vi "CountConfig.vi"(7 "Cal (F)/Acq (T) Counters":bool, 10 "Machine Type":enum16{"Hitachi", "B&K 3535", "B&K Hawk"}(ring), 11 "pulse delay  (cycles)":i16=1 caption="pulse delay (cycles)") -> (2 "task out":refnum<k21>)   [LabVIEW 2022 SP3]
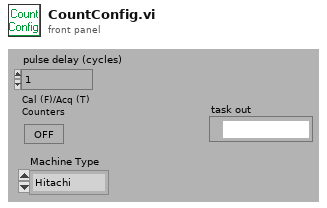
[diagram p1: front panel]
types:
  T1 = enum16{"gate on rising edge", "gate on falling edge"}
  T2 = enum16{"count on rising edge", "count on falling edge"}
  T3 = enum16{"arm on rising edge", "arm on falling edge"}
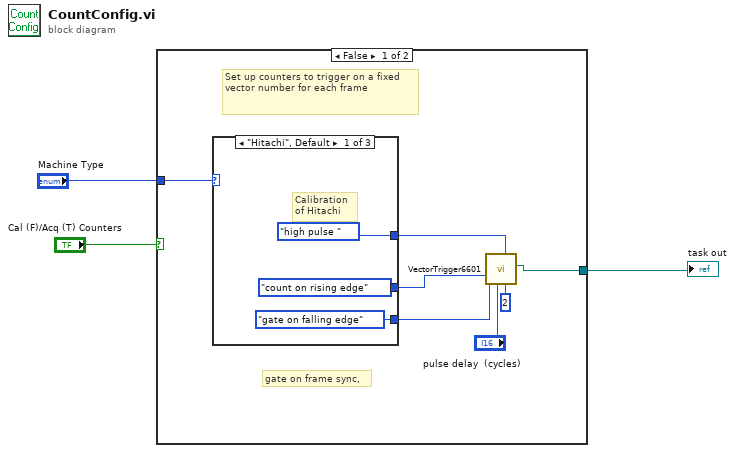
[diagram p0: block diagram]
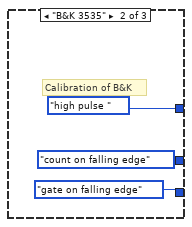
[diagram p2: hidden frame]
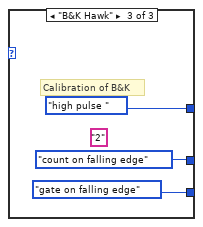
[diagram p3: hidden frame]
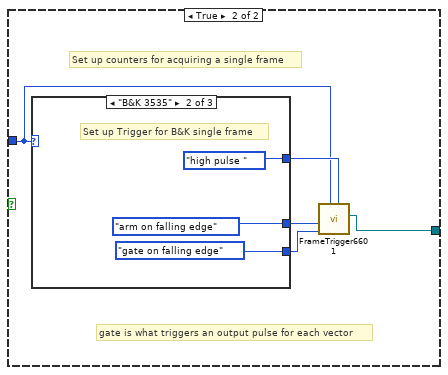
[diagram p4: hidden frame]
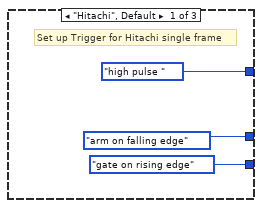
[diagram p5: hidden frame]
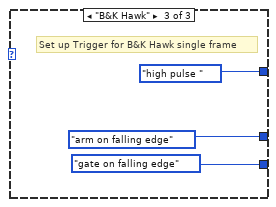
[diagram p6: hidden frame]
diagram:
  n1 = case shown="False" "Cal (F)/Acq (T) Counters" {
    tunnel: "Machine Type" -> [w5 w21]
    tunnel: [w4 w20] -> w1
    frame False {
      # "gate on frame sync,"
      # "Set up counters to trigger on a fixed vector number for each frame"
      n2 = case shown="\"Hitachi\", Default" w5 {
        tunnel: [enum16{"high pulse ", "low pulse"}."high pulse " ("pulse polarity (high:0)") enum16{"high pulse ", "low pulse"}."high pulse " ("pulse polarity (high:0)") enum16{"high pulse ", "low pulse"}."high pulse " ("pulse polarity (high:0)")] -> w8
        tunnel: [T2."count on rising edge" ("source edge") T2."count on falling edge" ("source edge") T2."count on falling edge" ("source edge")] -> w7
        tunnel: [T1."gate on falling edge" ("gate edge") T1."gate on falling edge" ("gate edge") T1."gate on falling edge" ("gate edge")] -> w6
        frame "Hitachi", Default {
          # "Calibration of Hitachi"
        }
        frame "B&K 3535" {
          # "Calibration of B&K"
        }
        frame "B&K Hawk" {
          (unwired) "2"
          # "Calibration of B&K"
        }
      }
      n3 = call "VectorTrigger6601.vi"("pulse width (cycles)"=2, "pulse polarity (high:0)"=w8, "pulse delay (cycles)"="pulse delay  (cycles)", "gate edge"=w6, "source edge"=w7) -> ("task out"=w4:refnum<k21>)  [unwired: 4 in, 2 out]
    }
    frame True {
      # "gate is what triggers an output pulse for each vector"
      # "Set up counters for acquiring a single frame"
      n4 = case shown="\"B&K 3535\"" w21 {
        tunnel: [enum16{"high pulse ", "low pulse"}."high pulse " ("pulse polarity (high:0)") enum16{"high pulse ", "low pulse"}."high pulse " ("pulse polarity (high:0)") enum16{"high pulse ", "low pulse"}."high pulse " ("pulse polarity (high:0)")] -> w24
        tunnel: [T1."gate on rising edge" ("gate edge") T1."gate on falling edge" ("gate edge") T1."gate on falling edge" ("gate edge")] -> w23
        tunnel: [T3."arm on falling edge" ("Trigger edge") T3."arm on falling edge" ("Trigger edge") T3."arm on falling edge" ("Trigger edge")] -> w22
        frame "Hitachi", Default {
          # "Set up Trigger for Hitachi single frame"
        }
        frame "B&K 3535" {
          # "Set up Trigger for B&K single frame"
        }
        frame "B&K Hawk" {
          # "Set up Trigger for B&K Hawk single frame"
        }
      }
      n5 = call "FrameTrigger6601.vi"("pulse polarity (high:0)"=w24, "Machine Type"=w21, "gate edge"=w23, "Counter Arm edge"=w22) -> ("task out"=w20:refnum<k21>)  [unwired: 4 in, 3 out]
    }
  }
  "task out" <- w1
